vi "Close Instrument.vi"(8 "error in (no error)":errorcluster, 11 "NI DMM.lvclass in":refnum<class "NI DMM.lvclass">) -> (0 "error out":errorcluster, 3 "NI DMM.lvclass out":refnum<class "NI DMM.lvclass">)   [LabVIEW 2011, in "NI DMM.lvclass"]
uses:
  NI DMM.lvclass
  NI DMM.lvclass/NI DMM.ctl
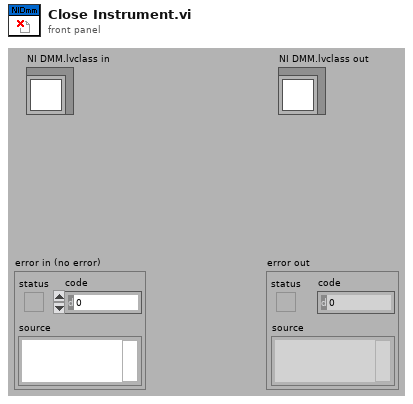
[diagram p1: front panel]
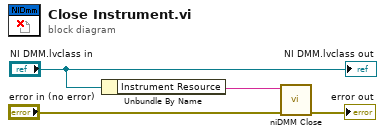
[diagram p0: block diagram]
diagram:
  n1 = Unbundle By Name("NI DMM.lvclass in") -> ("Instrument Resource"=w1:string)
  n2 = call <instrlib>:"niDMM Close.vi"("error in (no error)"="error in (no error)", "instrument handle"=w1) -> ("error out"=→"error out":errorcluster)  [unwired: 9 in]
  "NI DMM.lvclass out" <- "NI DMM.lvclass in"
